vi "Read functions.vi"(8 "error in":errorcluster, 11 "tag bus processing plugin module configuration in":refnum<class "tag bus processing plugin module configuration.lvclass">) -> (0 "error out":errorcluster, 2 "functions":T1[](array[typedef]), 3 "tag bus processing plugin module configuration out":refnum<class "tag bus processing plugin module configuration.lvclass">)   [LabVIEW 2013, in "tag bus processing plugin module configuration.lvclass"]
uses:
  tag bus processing plugin module configuration.lvclass
  processing channels.ctl
  <vilib>/NI/Tag Bus Module Framework/channel/TBM channel.lvclass
  tag bus processing plugin module configuration.lvclass/tag bus processing plugin module configuration.ctl
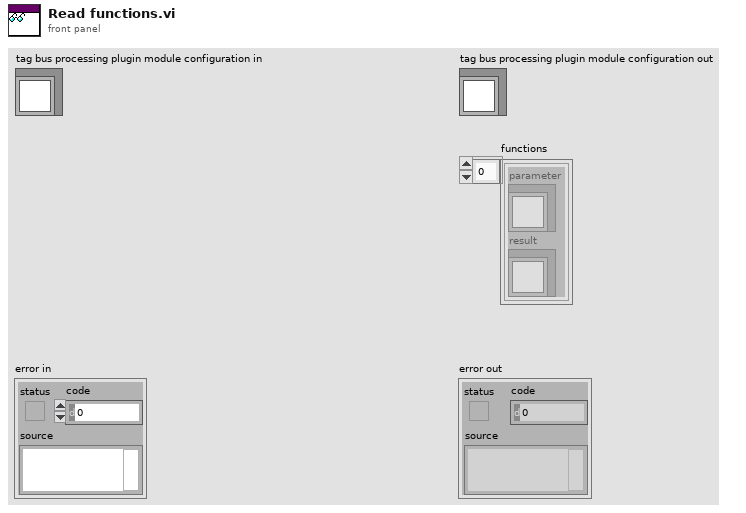
[diagram p1: front panel]
types:
  T1 = typedef "tag bus processing plugin module configuration.lvclass/processing channels.ctl" = cluster{"parameter":refnum<class "TBM channel.lvclass">, "result":refnum<class "TBM channel.lvclass">}
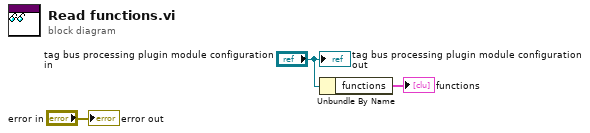
[diagram p0: block diagram]
diagram:
  n1 = Unbundle By Name("tag bus processing plugin module configuration in") -> ("functions"=→"functions":T1[])
  "error out" <- "error in"
  "tag bus processing plugin module configuration out" <- "tag bus processing plugin module configuration in"
